vi "Append Image.vi"(0 "PDF Report IN":refnum<class "PDF Report Class.lvclass">, 1 "Scale (%)":sgl=100.0, 3 "Border":T3={"Show?"=FALSE, "Thickness (point)"=0.5, "Color"=0}, 5 "Image path":path, 9 "Image Ref iTexSharp":refnum<k24>, 11 "error in (no error)":errorcluster, 12 "Caption":string, 14 "Position and indentation":T1={"Alignment"=enum."Center", "X "=0.0, "Y"=0.0, "Indentation"=0.0}) -> (4 "PDF Report OUT":refnum<class "PDF Report Class.lvclass">, 6 "Image path duplicate":path, 8 "Size (points)":cluster{"TotalHeight":sgl, "TotalWidth":sgl}, 15 "error out":errorcluster)   [LabVIEW 2019, in "Exaprom PDF.lvlib"]
doc: "The <B>VI</B> appends, to the PDF report, the image from a file. \n\nValid formats: GIF, JPEG, PNG and BMP.\n\n<B>FRANÇAIS</B>\nLe <B>VI</B> ajoute, au rapport PDF, l'image provenant d'un fichier.\n\nFormats valides : GIF, JPEG, PNG et BMP.\n\nVersion 1.0\nDeveloped by Jean-Marc Simard\nCopyright © 2010, Exaprom Inc.\nAll rights reserved.\nLicense: BSD\n\nWith iTextSharp 4.1.6 (http://itextsharp.sourceforge.net)\nunder Mozilla Public License Version 1.1\n(http://www.mozilla.org/MPL/MPL-1.1.html)"
uses:
  LV Class/PDF Report Class/PDF Report Class.lvclass
  C:/work/niobrara_lv/labview pdf writer fixing/DLL/itextsharp.dll
  DLL/itextsharp.dll
  Controls/Image Controls/Image border.ctl
  Controls/Image Controls/Image alignment and position.ctl
  Controls/Image Controls/Image aligment.ctl
  Controls/Image Controls/Image Scale Type.ctl
  Not  in the library/Images for controls/Image or Table.ctl
  Controls/Font Controls/Font complete cluster.ctl
  Controls/Font Controls/Font size.ctl
  Controls/Font Controls/Font color.ctl
  Controls/Font Controls/Type and encoding.ctl
  Controls/Text Controls/Unicode/Type and run direction.ctl
  Controls/Initialization Controls/Defaut Paragraphe and Line Spacing.ctl
  Controls/Text Controls/Line spacing.ctl
  Exaprom PDF.lvlib
  Controls/Text Controls/Texte alignement.ctl
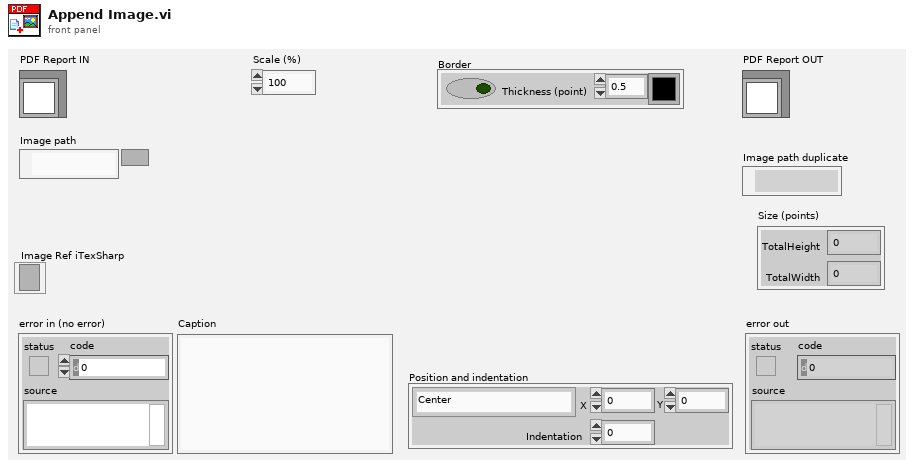
[diagram p1: front panel]
types:
  T1 = typedef "Exaprom PDF.lvlib/Image alignment and position.ctl" = cluster{"Alignment":T2, "X ":sgl, "Y":sgl, "Indentation":sgl}
  T2 = typedef "Exaprom PDF.lvlib/Image aligment.ctl" = enum16{"Absolute (X,Y)", "Left", "Center", "Right", "Left (textwrap)", "Right (textwrap)"}
  T3 = typedef "Exaprom PDF.lvlib/Image border.ctl" = cluster{"Show?":bool, "Thickness (point)":sgl, "Color":u32}
  T4 = typedef "Exaprom PDF.lvlib/Image Scale Type.ctl" = enum16{"%", "Height", "Width"}
  T5 = typedef "Exaprom PDF.lvlib/Image or Table.ctl" = enum16{"Image", "Table"}
  T6 = typedef "Exaprom PDF.lvlib/Defaut Paragraphe and Line Spacing.ctl" = cluster{" Aligment":T7, "Line spacing":T8}
  T7 = typedef "Exaprom PDF.lvlib/Texte alignement.ctl" = enum16{"Select", "CENTER", "JUSTIFY", "LEFT", "RIGHT"}
  T8 = typedef "Exaprom PDF.lvlib/Line spacing.ctl" = enum16{"Select", "1.0", "1.5", "2.0"}
  T9 = typedef "Exaprom PDF.lvlib/Font complete cluster.ctl" = cluster{"Name":string, "Size":T10, "Color":T11, "Style":cluster{"Bold":bool, "Italic":bool, "Underline":bool, "Strikeout":bool}, "Type":T12}
  T10 = typedef "Exaprom PDF.lvlib/Font size.ctl" = sgl
  T11 = typedef "Exaprom PDF.lvlib/Font color.ctl" = u32
  T12 = typedef "Exaprom PDF.lvlib/Type and encoding.ctl" = cluster{"Type&direction":T13, "Embedded":bool, "Encoding":string}
  T13 = typedef "Exaprom PDF.lvlib/Type and run direction.ctl" = enum16{"Select", "ASCII", "UTF-16", "UTF-16 (default)", "UTF-16 (LTR)", "UTF-16 (RTL)"}
  T14 = typedef "Exaprom PDF.lvlib/Unit.ctl" = enum16{"inch", "mm"}
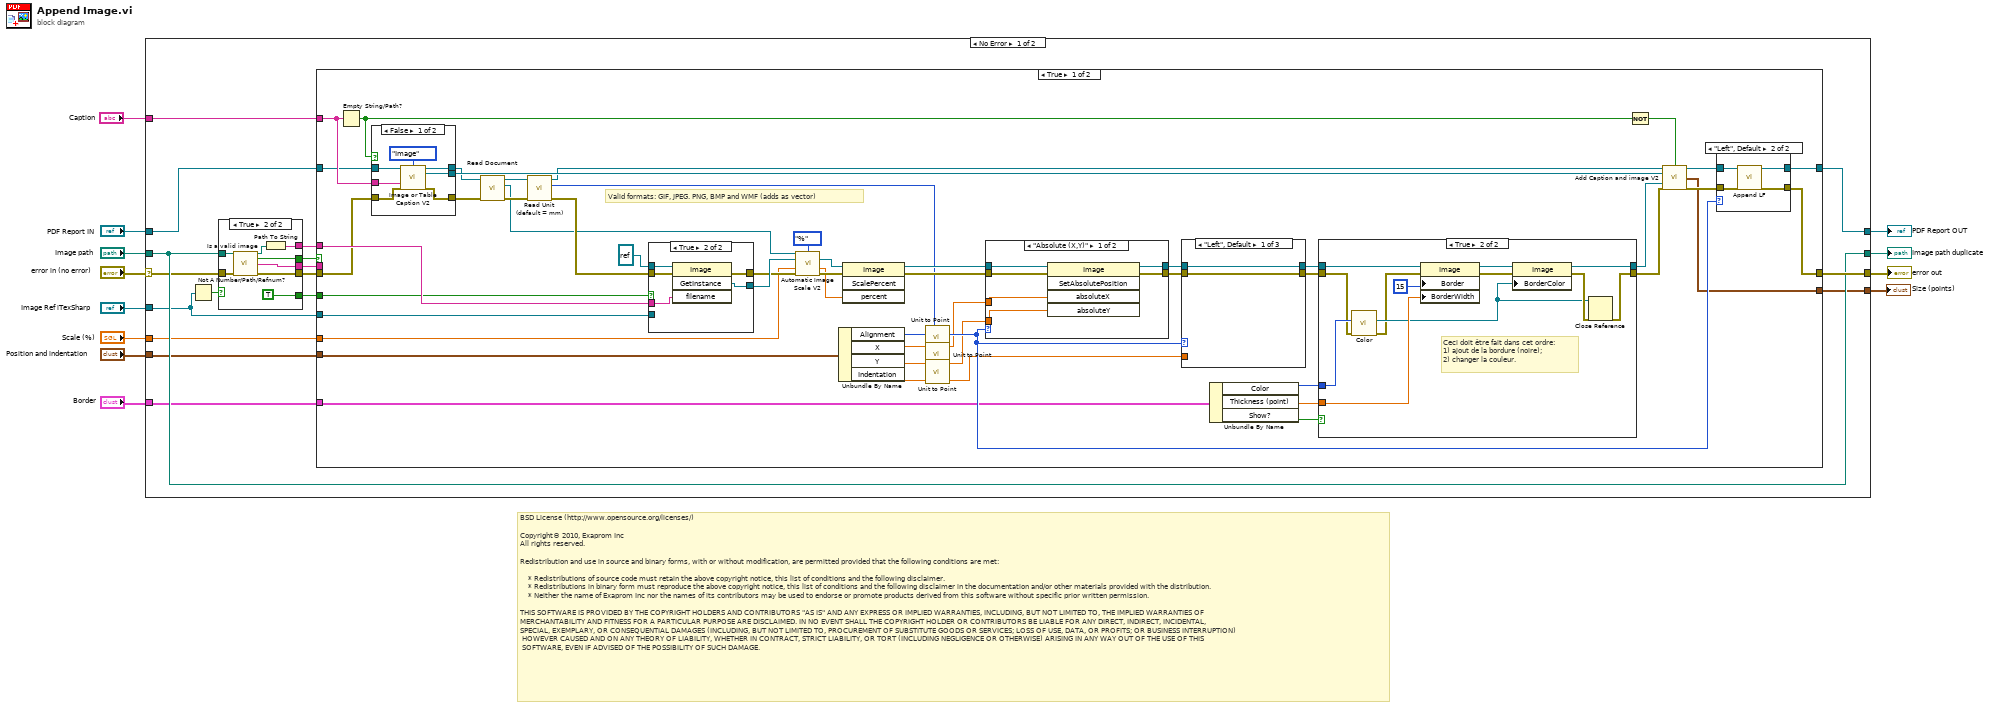
[diagram p0: block diagram]
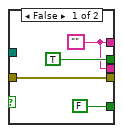
[diagram p2: hidden frame]
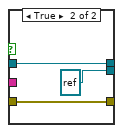
[diagram p5: hidden frame]
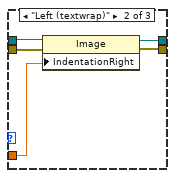
[diagram p6: hidden frame]
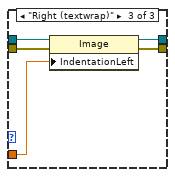
[diagram p7: hidden frame]
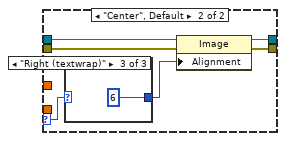
[diagram p9: hidden frame]
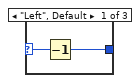
[diagram p10: hidden frame]
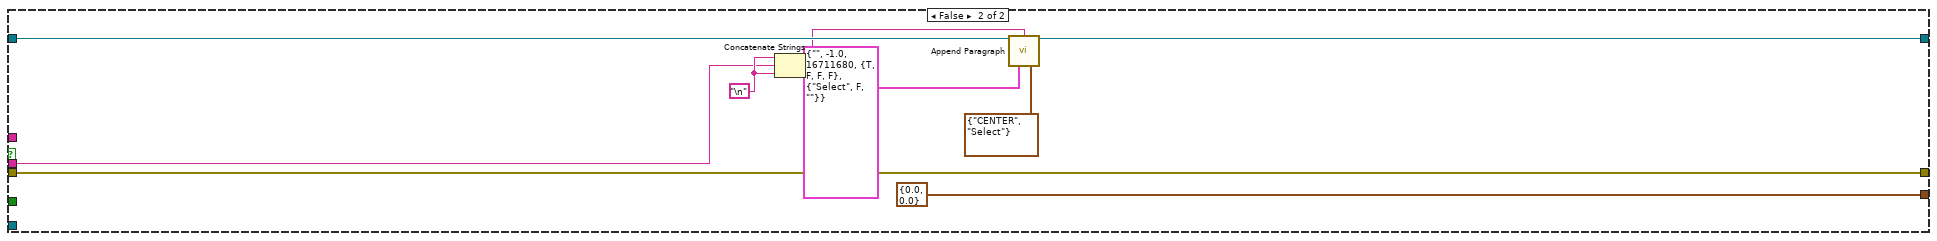
[diagram p12: hidden frame]
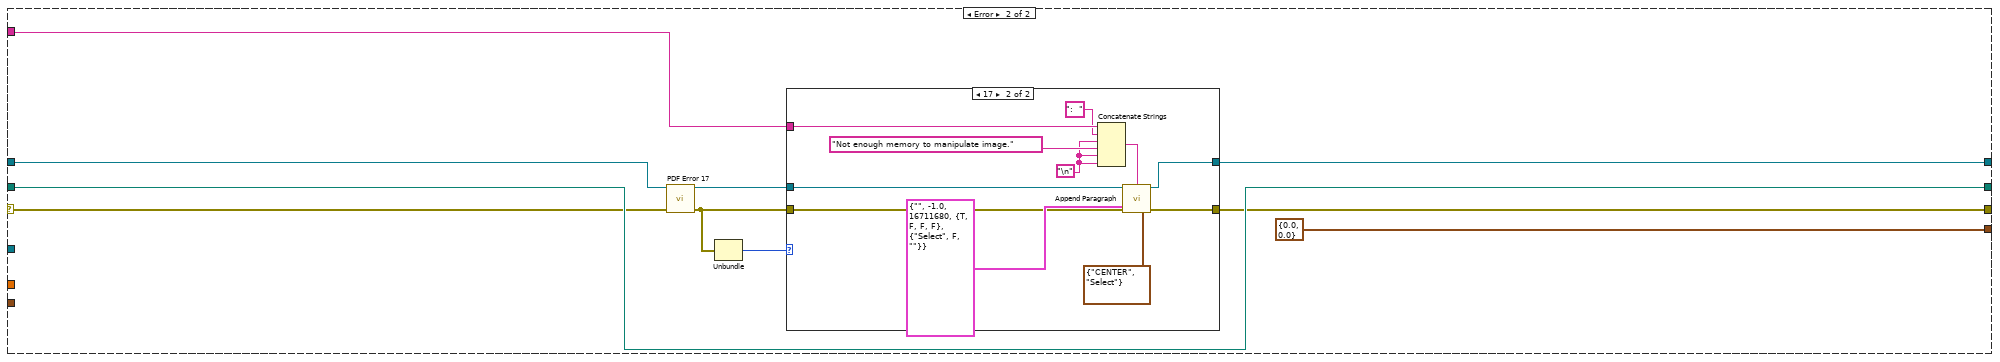
[diagram p13: hidden frame]
diagram:
  # "BSD License (http://www.opensource.org/licenses/)\n\nCopyright© 2010, Exaprom Inc\nAll rights reserved.\n\nRedistribution and use in source and binary forms, with or without modification, are permitted provided that the following conditions are met:\n\n    * Redistributions of source code must retain the above copyright notice, this list of conditions and the following disclaimer.\n    * Redistributions in binary form must reproduce the above copyright notice, this list of conditions and the following disclaimer in the documentation and/or other materials provided with the distribution.\n    * Neither the name of Exaprom Inc nor the names of its contributors may be used to endorse or promote products derived from this software without specific prior written permission.\n\nTHIS SOFTWARE IS PROVIDED BY THE COPYRIGHT HOLDERS AND CONTRIBUTORS \"AS IS\" AND ANY EXPRESS OR IMPLIED WARRANTIES, INCLUDING, BUT NOT LIMITED TO, THE IMPLIED WARRANTIES OF \nMERCHANTABILITY AND FITNESS FOR A PARTICULAR PURPOSE ARE DISCLAIMED. IN NO EVENT SHALL THE COPYRIGHT HOLDER OR CONTRIBUTORS BE LIABLE FOR ANY DIRECT, INDIRECT, INCIDENTAL,\nSPECIAL, EXEMPLARY, OR CONSEQUENTIAL DAMAGES (INCLUDING, BUT NOT LIMITED TO, PROCUREMENT OF SUBSTITUTE GOODS OR SERVICES; LOSS OF USE, DATA, OR PROFITS; OR BUSINESS INTERRUPTION)\n HOWEVER CAUSED AND ON ANY THEORY OF LIABILITY, WHETHER IN CONTRACT, STRICT LIABILITY, OR TORT (INCLUDING NEGLIGENCE OR OTHERWISE) ARISING IN ANY WAY OUT OF THE USE OF THIS\n SOFTWARE, EVEN IF ADVISED OF THE POSSIBILITY OF SUCH DAMAGE."
  n1 = case shown="No Error" "error in (no error)" {
    selector: "error in (no error)" -> [w14 w172]
    tunnel: [w22 w168] -> w7
    tunnel: [w29 w167] -> w12
    tunnel: "PDF Report IN" -> [w24 w173]
    tunnel: "Image path" -> [w25 w174]
    tunnel: [w25 w174] -> w9
    tunnel: "Caption" -> [w23 w166]
    tunnel: "Image Ref iTexSharp" -> [w19 _]
    tunnel: "Border" -> [w18 _]
    tunnel: "Position and indentation" -> [w17 _]
    tunnel: "Scale (%)" -> [w16 _]
    tunnel: [w15 cluster{"TotalHeight":sgl, "TotalWidth":sgl} {"TotalHeight"=0.0, "TotalWidth"=0.0}] -> w1
    frame No Error {
      n2 = Not A Number/Path/Refnum?(number/path/refnum=w19) -> (NaN/Path/Refnum?=w21:bool)
      n3 = case shown="True" w21 {
        tunnel: [w31 w40] -> w28
        tunnel: [TRUE ("Valid Image?") w35] -> w27
        tunnel: [w30 w39] -> w26
        tunnel: w25 -> [_ w38]
        tunnel: [FALSE TRUE] -> w20
        tunnel: w14 -> [w30 w36]
        tunnel: [w31 w34] -> w13
        frame False {
          w31 = ""
        }
        frame True {
          n4 = call "Is a valid image.vi"("Image path"=w38, "error in (no error)"=w36) -> ("dup path"=w41:path, "Valid Image?"=w35:bool, "Message"=w34:string, "error out"=w39:errorcluster)  [unwired: 10 out]
          n5 = Path To String(path=w41) -> (string=w40:string)
        }
      }
      n6 = case shown="True" w27 {
        tunnel: [w62 w158] -> w29
        tunnel: w28 -> [w87 _]
        tunnel: w26 -> [w60 w158]
        tunnel: w24 -> [w64 w165]
        tunnel: w23 -> [w75 _]
        tunnel: [w63 w163] -> w22
        tunnel: w20 -> [w74 _]
        tunnel: w19 -> [w73 _]
        tunnel: w18 -> [w72 _]
        tunnel: w17 -> [w70 _]
        tunnel: w16 -> [w51 _]
        tunnel: [w53 cluster{"TotalHeight":sgl, "TotalWidth":sgl} {"TotalHeight"=0.0, "TotalWidth"=0.0}] -> w15
        tunnel: w13 -> [_ w157]
        frame True {
          # "Valid formats: GIF, JPEG. PNG, BMP and WMF (adds as vector)"
          n7 = Empty String/Path?(string/path=w75) -> (empty?=w58:bool)
          n8 = case shown="False" w58 {
            tunnel: [w111 w114] -> w44
            tunnel: w64 -> [w110 w114]
            tunnel: w75 -> [w109 _]
            tunnel: [w108 w113] -> w76
            tunnel: [w107 refnum<k24> refnum ("Paragraph Refnum")] -> w55
            tunnel: w60 -> [w106 w113]
            frame False {
              n9 = call "Image or Table Caption V2.vi"("PDF Report IN"=w110, "Image or Table"=Image_or_Table."Image", "Caption IN"=w109, "error IN"=w106) -> ("PDF Report OUT"=w111:refnum<class "PDF Report Class.lvclass">, "PdfpTable Refnum"=w107:refnum<k24>, "error OUT"=w108:errorcluster)  [unwired: 4 in, 5 out]
            }
            frame True {
              (unwired) sgl 2.0 ("Largeur (default unit)")
              (unwired) u32 0
              (unwired) refnum<k24> refnum ("Cell ref")
              (unwired) sgl 0.0 ("TotalHeight")
            }
          }
          n10 = call-dynamic "Read Document.vi"("error in (no error)"=w76, "PDF Report Class in"=w44) -> ("error out"=w49:errorcluster, "Document"=w46:refnum<k24>, "PDF Report Class out"=w43:refnum<class "PDF Report Class.lvclass">)  [unwired: 7 in]
          n11 = call-dynamic "Read Unit (default = mm).vi"("error in (no error)"=w49, "PDF Report Class in"=w43) -> ("error out"=w48:errorcluster, "Unit (default = mm)"=w47:T14, "PDF Report Class out"=w45:refnum<class "PDF Report Class.lvclass">)  [unwired: 7 in]
          n12 = case shown="True" w74 {
            tunnel: refnum<k24> refnum ("image") -> [_ w104]
            tunnel: w87 -> [_ w103]
            tunnel: [w98 w102] -> w84
            tunnel: [w99 w101] -> w82
            tunnel: w48 -> [w99 w100]
            tunnel: w73 -> [w98 _]
            frame False {
            }
            frame True {
              n13 = invoke class="Image" method="GetInstance"(reference=w104, error in=w100, "filename"=w103) -> (error out=w101:errorcluster, "GetInstance"=w102:refnum<k24>)  [unwired: 1 in, 2 out]
            }
          }
          n14 = call "Automatic Image Scale V2.vi"("Document"=w46, "Scale Type"=Image_Scale_Type."%", "GetInstanceImage IN"=w84, "Scale percent IN"=w51, "error in (no error)"=w82) -> ("GetInstanceImage OUT"=w83:refnum<k24>, "Scale percent OUT"=w80:sgl, "error out"=w81:errorcluster)  [unwired: 6 in, 2 out]
          n15 = Unbundle By Name(w70) -> ("Alignment"=w91:T2, "X"=w67:sgl, "Y"=w68:sgl, "Indentation"=w69:sgl)
          n16 = invoke class="Image" method="ScalePercent"(reference=w83, error in=w81, "percent"=w80) -> (reference out=w89:refnum<k24>, error out=w90:errorcluster)  [unwired: 1 in, 2 out]
          n17 = call "Unit to Point.vi"("X unit"=w67, "Unit (default = mm)"=w47) -> ("X point"=w86:sgl)  [unwired: 7 out]
          n18 = call "Unit to Point.vi"("X unit"=w68, "Unit (default = mm)"=w47) -> ("X point"=w85:sgl)  [unwired: 7 out]
          n19 = call "Unit to Point.vi"("X unit"=w69, "Unit (default = mm)"=w47) -> ("X point"=w50:sgl)  [unwired: 7 out]
          n20 = case shown="\"Absolute (X,Y)\"" w91 {
            selector: w91 -> [_ w147]
            tunnel: [w146 w152] -> w78
            tunnel: [w145 w149] -> w77
            tunnel: w90 -> [w144 w150]
            tunnel: w89 -> [w143 w151]
            tunnel: w86 -> [w142 _]
            tunnel: w85 -> [w141 _]
            frame "Absolute (X,Y)" {
              n21 = invoke class="Image" method="SetAbsolutePosition"(reference=w143, error in=w144, "absoluteX"=w142, "absoluteY"=w141) -> (reference out=w146:refnum<k24>, error out=w145:errorcluster)  [unwired: 1 in, 3 out]
            }
            frame "Center", Default {
              n22 = case shown="\"Right (textwrap)\"" w147 {
                selector: w147 -> [w153 w155 _]
                tunnel: [w154 w155 6] -> w148
                frame "Left", Default {
                  n23 = Decrement(x=w153) -> (x-1=w154:T2)
                }
                frame "Left (textwrap)" {
                }
                frame "Right (textwrap)" {
                }
              }
              n24 = property class="Image"(reference=w151, error in=w150, "Alignment"=w148) -> (reference out=w152:refnum<k24>, error out=w149:errorcluster)
            }
          }
          n25 = case shown="\"Left\", Default" w91 {
            tunnel: [w116 w118 w126] -> w79
            tunnel: w78 -> [w116 w121 w123]
            tunnel: [w115 w119 w125] -> w66
            tunnel: w77 -> [w115 w120 w124]
            tunnel: w50 -> [_ w117 w122]
            frame "Left", Default {
            }
            frame "Left (textwrap)" {
              n26 = property class="Image"(reference=w121, error in=w120, "IndentationRight"=w117) -> (reference out=w118:refnum<k24>, error out=w119:errorcluster)
            }
            frame "Right (textwrap)" {
              n27 = property class="Image"(reference=w123, error in=w124, "IndentationLeft"=w122) -> (reference out=w126:refnum<k24>, error out=w125:errorcluster)
            }
          }
          n28 = Unbundle By Name(w72) -> ("Color"=w61:u32, "Thickness (point)"=w65:sgl, "Show?"=w71:bool)
          n29 = case shown="True" w71 {
            tunnel: w79 -> [w128 w137]
            tunnel: [w128 w138] -> w56
            tunnel: [w127 w135] -> w57
            tunnel: w66 -> [w127 w130]
            tunnel: w61 -> [_ w132]
            tunnel: w65 -> [_ w134]
            frame False {
            }
            frame True {
              # "Ceci doit être fait dans cet ordre:\n1) ajout de la bordure (noire);\n2) changer la couleur."
              n30 = call "Color.vi"("error in (no error)"=w130, "Color"=w132) -> ("error out"=w129:errorcluster, "Color"=w131:refnum<k24>)  [unwired: 8 out]
              n31 = property class="Image"(reference=w137, error in=w129, "Border"=15, "BorderWidth"=w134) -> (reference out=w133:refnum<k24>, error out=w139:errorcluster)
              n32 = property class="Image"(reference=w133, error in=w139, "BorderColor"=w131) -> (reference out=w138:refnum<k24>, error out=w136:errorcluster)
              n33 = Close Reference(reference=w131, error in (no error)=w136) -> (error out=w135:errorcluster)
            }
          }
          n34 = Not(x=w58) -> (.not. x?=w52:bool)
          n35 = call "Add Caption and image V2.vi"("PDF Report IN"=w45, "Caption?"=w52, "Paragraph Refnum"=w55, "Image Ref iTexSharp"=w56, "error in (no error)"=w57) -> ("PDF Report OUT"=w59:refnum<class "PDF Report Class.lvclass">, "Size (points)"=w53:cluster{"TotalHeight":sgl, "TotalWidth":sgl}, "error out"=w54:errorcluster)  [unwired: 8 out]
          n36 = case shown="\"Left\", Default" w91 {
            tunnel: w59 -> [w92 w97]
            tunnel: [w92 w96] -> w63
            tunnel: [w93 w95] -> w62
            tunnel: w54 -> [w93 w94]
            frame "Left (textwrap)", "Right (textwrap)" {
            }
            frame "Left", Default {
              n37 = call "Append LF.vi"("PDF Report IN"=w97, "error in (no error)"=w94) -> ("PDF Report duplicate"=w96:refnum<class "PDF Report Class.lvclass">, "error out"=w95:errorcluster)  [unwired: 2 in, 10 out]
            }
          }
        }
        frame False {
          w162 = "\n"
          n38 = Concatenate Strings(w162, w157, w162) -> (w161:string)
          n39 = call "Append Paragraph.vi"("PDF Report"=w165, "Text"=w161, "Font"=T9 {"Name"="", "Size"=-1.0, "Color"=16711680, "Style"={"Bold"=TRUE, "Italic"=FALSE, "Underline"=FALSE, "Strikeout"=FALSE}, "Type"={"Type&direction"=enum."Select", "Embedded"=FALSE, "Encoding"=""}} ("Font complete"), "Paragraph properties"=T6 {" Aligment"=enum."CENTER", "Line spacing"=enum."Select"}) -> ("PDF Report duplicate"=w163:refnum<class "PDF Report Class.lvclass">)  [unwired: 4 in, 7 out]
        }
      }
    }
    frame Error {
      n40 = call "PDF Error 17.vi"("PDF Report IN"=w173, "error in (no error)"=w172) -> ("PDF Report OUT"=w169:refnum<class "PDF Report Class.lvclass">, "error out"=w170:errorcluster)  [unwired: 12 out]
      n41 = Unbundle(w170) -> ("code"=w171:i32)  [unwired: 2 out]
      n42 = case shown="17" w171 {
        tunnel: w170 -> [w176 w185]
        tunnel: w169 -> [w177 w184]
        tunnel: [w177 w183] -> w168
        tunnel: [w176 w182] -> w167
        tunnel: w166 -> [_ w179]
        frame 0, Default {
        }
        frame 17 {
          w180 = "\n"
          n43 = Concatenate Strings(w179, ":  ", w180, "Not enough memory to manipulate image.", w180, w180) -> (w188:string)
          n44 = call "Append Paragraph.vi"("PDF Report"=w184, "Text"=w188, "error in (no error)"=w185, "Font"=T9 {"Name"="", "Size"=-1.0, "Color"=16711680, "Style"={"Bold"=TRUE, "Italic"=FALSE, "Underline"=FALSE, "Strikeout"=FALSE}, "Type"={"Type&direction"=enum."Select", "Embedded"=FALSE, "Encoding"=""}} ("Font complete"), "Paragraph properties"=T6 {" Aligment"=enum."CENTER", "Line spacing"=enum."Select"}) -> ("PDF Report duplicate"=w183:refnum<class "PDF Report Class.lvclass">, "error out"=w182:errorcluster)  [unwired: 3 in, 6 out]
        }
      }
    }
  }
  "error out" <- w12
  "PDF Report OUT" <- w7
  "Image path duplicate" <- w9
  "Size (points)" <- w1
